vi "质控启动流程对话框.vi"() -> (0 "确定启动":bool, 1 "启动模块":cluster{"氨氮1":bool, "总磷1":bool, " COD1":bool}, 2 "直接启动":bool, 3 "常规启动":bool)   [LabVIEW 2016, in "质控单元.lvlib"]
panel:
  in  "直接启动":bool
  in  "取消":bool
  in  "常规启动":bool
  # "请选择启动模式"
  # "常规启动：先启动采配水，再进行加标回收"
  # "直接启动：不启动采配水，直接加标回收"
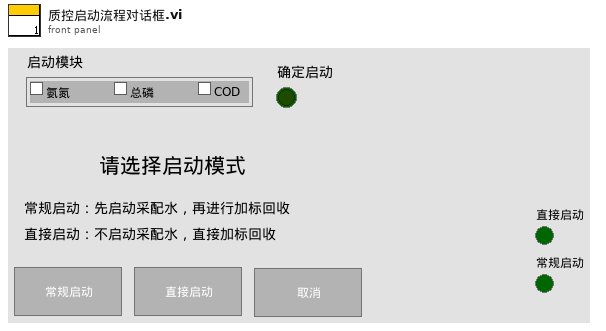
[diagram p1: front panel]
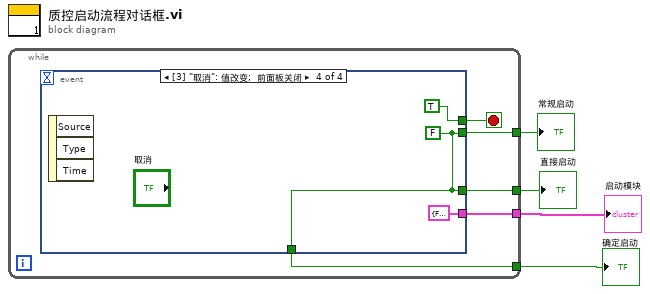
[diagram p0: block diagram]
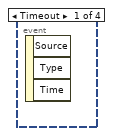
[diagram p2: hidden frame]
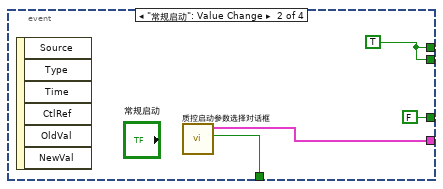
[diagram p3: hidden frame]
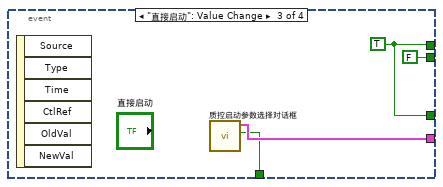
[diagram p4: hidden frame]
diagram:
  n1 = while {
    tunnel: [w8] -> w4
    tunnel: [w7] -> w3
    tunnel: [w6] -> w2
    tunnel: [w5] -> w1
    stop <- w9 stop-if-true
    n2 = event shown="[3] \"取消\": 值改变;  前面板关闭" {
      selector: _ -> [_ _ _ _]
      dyn-events: _ -> [_ _ _ _]
      timeout: _ -> [_ _ _ _]
      tunnel: [_ w13 w17 TRUE ("确定")] -> w9
      tunnel: [_ w13 FALSE ("确定") w19] -> w8
      tunnel: [_ FALSE ("确定") w17 w19] -> w7
      tunnel: [_ w11 w15 cluster{"氨氮1":bool, "总磷1":bool, " COD1":bool} {"氨氮1"=FALSE, "总磷1"=FALSE, " COD1"=FALSE} ("启动模块")] -> w6
      tunnel: [_ w10 w14 w19] -> w5
      event Timeout {
        n3 = event-data() -> ()  [unwired: 1 in, 3 out]
      }
      event "常规启动": Value Change {
        w13 = TRUE ("确定")
        n4 = event-data() -> ()  [unwired: 1 in, 6 out]
        n5 = call "质控启动参数选择对话框.vi"() -> ("确定启动"=w10:bool, "启动模块"=w11:cluster{"氨氮1":bool, "总磷1":bool, " COD1":bool})  [unwired: 9 in, 1 out]
      }
      event "直接启动": Value Change {
        w17 = TRUE ("确定")
        n6 = event-data() -> ()  [unwired: 1 in, 6 out]
        n7 = call "质控启动参数选择对话框.vi"() -> ("确定启动"=w14:bool, "启动模块"=w15:cluster{"氨氮1":bool, "总磷1":bool, " COD1":bool})  [unwired: 9 in, 1 out]
      }
      event "取消": Value Change; Panel Close {
        w19 = FALSE ("确定")
        n8 = event-data() -> ()  [unwired: 1 in, 3 out]
      }
    }
  }
  "常规启动" <- w4
  "直接启动" <- w3
  "启动模块" <- w2
  "确定启动" <- w1
